vi "NormalizeMaxMin.vi"(1 "Min":sgl, 2 "Max":sgl, 3 "Score":sgl[](array[numeric])) -> (0 "Array":sgl[](array[numeric]))   [LabVIEW 2014]
panel:
  # "LICENSED MATERIALS – PROPERTY OF IBM\nCopyright IBM Corp. 2016, 2016\nALL RIGHTS RESERVED"
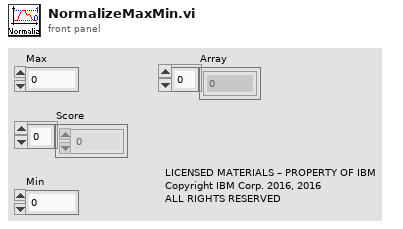
[diagram p1: front panel]
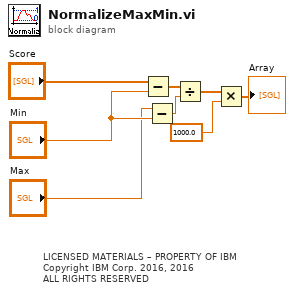
[diagram p0: block diagram]
diagram:
  # "LICENSED MATERIALS – PROPERTY OF IBM\nCopyright IBM Corp. 2016, 2016\nALL RIGHTS RESERVED"
  n1 = Subtract(x="Score", y="Min") -> (x-y=w2:sgl[])
  n2 = Subtract(x="Max", y="Min") -> (x-y=w1:sgl)
  n3 = Divide(x=w2, y=w1) -> (x/y=w7:sgl[])
  n4 = Multiply(x=w7, y=sgl 1000.0 ("x-y")) -> (x*y=→"Array":sgl[])
